vi "test Set and Get Properties.vi"(8 "error in (no error)":errorcluster, 11 "TestCase in":refnum<class "SLSC Switch Scripting Unit Tests.lvclass">) -> (0 "error out":errorcluster, 3 "TestCase out":refnum<class "SLSC Switch Scripting Unit Tests.lvclass">)   [LabVIEW 2017, in "SLSC Switch Scripting Unit Tests.lvclass"]
uses:
  SLSC Switch Scripting Unit Tests.lvclass
  Properties/SLSC Switch All Properties.ctl
  SLSC Switch Scripting Unit Tests.lvclass/SLSC Switch Scripting Unit Tests.ctl
  <vilib>/addons/_JKI Toolkits/VI Tester/TestCase.llb/TestCase.lvclass
  SLSC Switch Scripting.lvlib
  C:/Program Files (x86)/National Instruments/LabVIEW 2017/vi.lib/addons/_JKI Toolkits/VI Tester/TestCase.llb/TestCase.lvclass
panel:
  in  "Save?":bool
  out "Output Filename":string
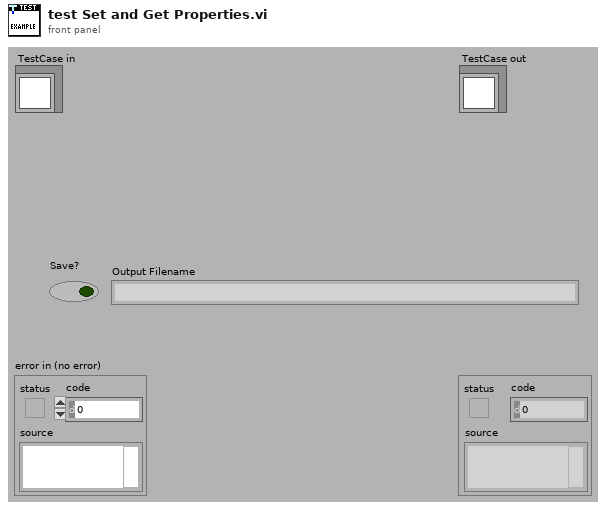
[diagram p1: front panel]
types:
  T1 = typedef "SLSC Switch Scripting.lvlib/SLSC Switch All Properties.ctl" = cluster{"Model":string, "Resource":string, "Topology":string, "Capabilities Version":string, "Capabilities":string}
  T2 = typedef "Custom Device API.lvlib/Custom Device Item Ref.ctl" = u64
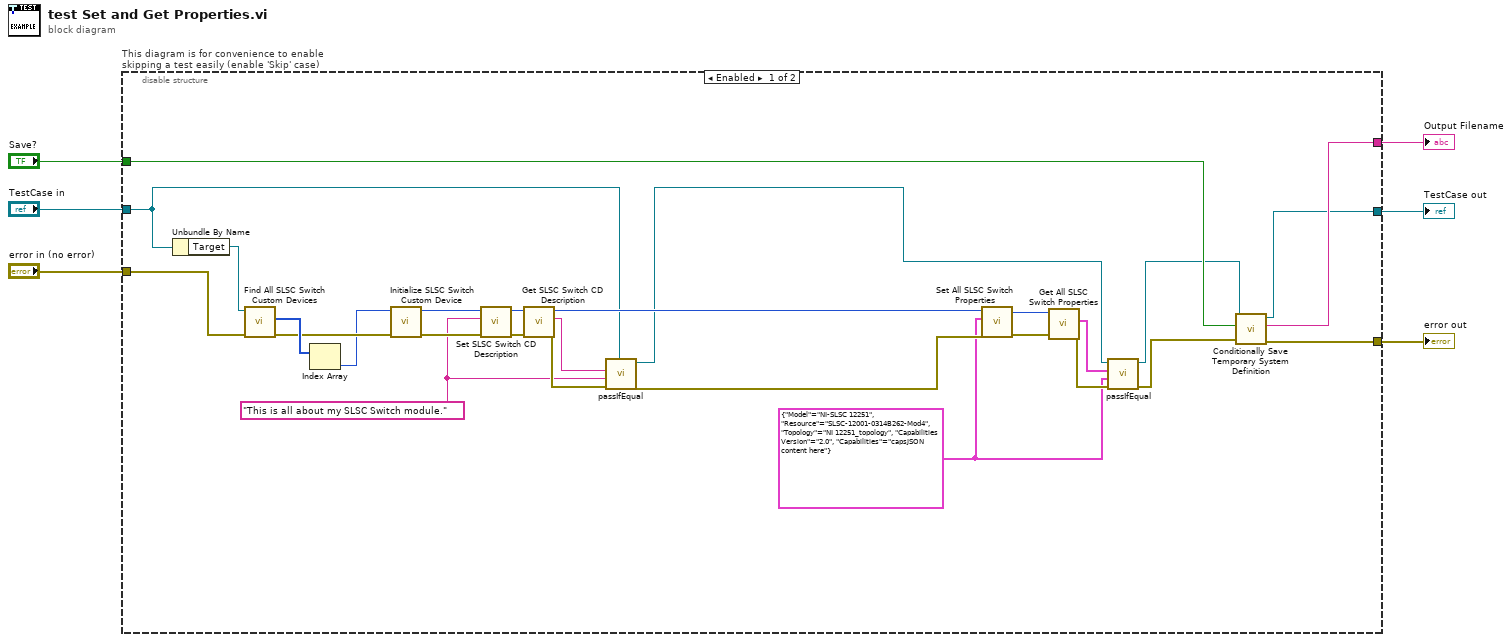
[diagram p0: block diagram]
diagram:
  n1 = disable-structure "This diagram is for convenience to enable skipping a test easily (enable 'Skip' case)" shown="Enabled" {
    disable-tunnel: "TestCase in" -> [w17 w37]
    disable-tunnel: [w31 w35] -> w3
    disable-tunnel: [w32 w36] -> w5
    disable-tunnel: "error in (no error)" -> [w25 w34]
    disable-tunnel: [w33 _] -> w2
    disable-tunnel: "Save?" -> [w30 _]
    frame Enabled {
      w7 = T1 {"Model"="NI-SLSC 12251", "Resource"="SLSC-12001-0314B262-Mod4", "Topology"="NI 12251_topology", "Capabilities Version"="2.0", "Capabilities"="capsJSON content here"} ("SLSC Switch All Properties")
      w12 = "This is all about my SLSC Switch module." ("Description")
      n2 = Unbundle By Name(w17) -> ("Target"=w26:refnum<k24>)
      n3 = call "Find All SLSC Switch Custom Devices.vi"("error in (no error)"=w25, "Target in"=w26) -> ("error out"=w28:errorcluster, "SLSC Switch Custom Device Ref IDs"=w29:T2[])  [unwired: 7 in, 1 out]
      n4 = Index Array(array=w29) -> (element=w27:T2)  [unwired: 1 in]
      n5 = call "Initialize SLSC Switch Custom Device.vi"("error in (no error)"=w28, "SLSC Sw Custom Device Ref in"=w27) -> ("error out"=w21:errorcluster, "SLSC Sw Custom Device Ref out"=w22:T2)  [unwired: 7 in, 1 out]
      n6 = call "Set SLSC Switch CD Description.vi"("error in (no error)"=w21, "Description"=w12, "SLSC Sw Custom Device Ref in"=w22) -> ("error out"=w14:errorcluster, "SLSC Sw Custom Device Ref out"=w20:T2)  [unwired: 7 in]
      n7 = call "Get SLSC Switch CD Description.vi"("error in (no error)"=w14, "SLSC Sw Custom Device Ref in"=w20) -> ("error out"=w15:errorcluster, "Description"=w18:string, "SLSC Sw Custom Device Ref out"=w19:T2)  [unwired: 7 in]
      n8 = call-dynamic "passIfEqual.vi"("error in (no error)"=w15, "y"=w12, "x"=w18, "TestCase in"=w17) -> ("error out"=w13:errorcluster, "TestCase out"=w16:refnum<class "SLSC Switch Scripting Unit Tests.lvclass">)  [unwired: 6 in]
      n9 = call "Set All SLSC Switch Properties.vi"("error in (no error)"=w13, "SLSC Switch All Properties"=w7, "SLSC Sw Custom Device Ref in"=w19) -> ("error out"=w8:errorcluster, "SLSC Sw Custom Device Ref out"=w9:T2)  [unwired: 7 in]
      n10 = call "Get All SLSC Switch Properties.vi"("error in (no error)"=w8, "SLSC Sw Custom Device Ref in"=w9) -> ("error out"=w11:errorcluster, "SLSC Switch All Properties"=w10:T1)  [unwired: 7 in, 1 out]
      n11 = call-dynamic "passIfEqual.vi"("error in (no error)"=w11, "y"=w7, "x"=w10, "TestCase in"=w16) -> ("error out"=w23:errorcluster, "TestCase out"=w24:refnum<class "SLSC Switch Scripting Unit Tests.lvclass">)  [unwired: 6 in]
      n12 = call "Conditionally Save Temporary System Definition.vi"("error in (no error)"=w23, "Save?"=w30, "Test Case"=w24) -> ("error out"=w32:errorcluster, "filename"=w33:string, "Test Case"=w31:refnum<class "SLSC Switch Scripting Unit Tests.lvclass">)  [unwired: 6 in]
    }
    frame Disabled {
      # "skip test result while test is under development"
      n13 = call <vilib>:"skip.vi"("error in (no error)"=w34, "TestCase in"=w37) -> ("error out"=w36:errorcluster, "TestCase out"=w35:refnum<class "SLSC Switch Scripting Unit Tests.lvclass">)  [unwired: 8 in]
    }
  }
  "error out" <- w5
  "TestCase out" <- w3
  "Output Filename" <- w2
